vi "Line Intersection.vi"(4 "y 4":dbl, 5 "x 1":dbl, 6 "x 4":dbl, 7 "y 1":dbl, 8 "y 3":dbl, 9 "x 3":dbl, 10 "y 2":dbl, 11 "x 2":dbl) -> (2 "y":dbl, 3 "x":dbl)   [LabVIEW 2020, in "NI_AAL_Geometry.lvlib"]
uses:
  <vilib>/Analysis/NI_AAL_Geometry.lvlib
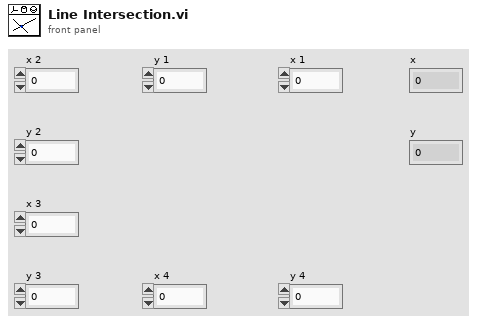
[diagram p1: front panel]
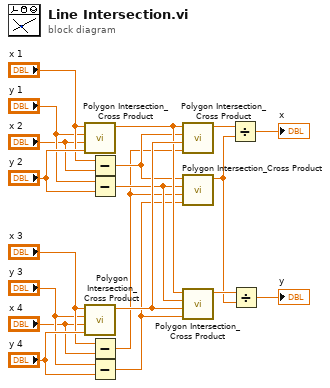
[diagram p0: block diagram]
diagram:
  n1 = call <vilib>:"Polygon Intersection_Cross Product.vi"("y 2"="y 2", "x 2"="x 2", "y 1"="y 1", "x 1"="x 1") -> ("Corss Product"=w12:dbl)  [unwired: 7 in]
  n2 = call <vilib>:"Polygon Intersection_Cross Product.vi"("y 2"="y 4", "x 2"="x 4", "y 1"="y 3", "x 1"="x 3") -> ("Corss Product"=w13:dbl)  [unwired: 7 in]
  n3 = Subtract(x="x 1", y="x 2") -> (x-y=w4:dbl)
  n4 = Subtract(x="y 1", y="y 2") -> (x-y=w3:dbl)
  n5 = Subtract(x="x 3", y="x 4") -> (x-y=w2:dbl)
  n6 = Subtract(x="y 3", y="y 4") -> (x-y=w1:dbl)
  n7 = call <vilib>:"Polygon Intersection_Cross Product.vi"("y 2"=w2, "x 2"=w13, "y 1"=w4, "x 1"=w12) -> ("Corss Product"=w11:dbl)  [unwired: 7 in]
  n8 = call <vilib>:"Polygon Intersection_Cross Product.vi"("y 2"=w1, "x 2"=w2, "y 1"=w3, "x 1"=w4) -> ("Corss Product"=w8:dbl)  [unwired: 7 in]
  n9 = call <vilib>:"Polygon Intersection_Cross Product.vi"("y 2"=w1, "x 2"=w13, "y 1"=w3, "x 1"=w12) -> ("Corss Product"=w9:dbl)  [unwired: 7 in]
  n10 = Divide(x=w11, y=w8) -> (x/y=→"x":dbl)
  n11 = Divide(x=w9, y=w8) -> (x/y=→"y":dbl)
